vi "Load Positions.vi"(8 "error in":errorcluster) -> (0 "error out":errorcluster, 3 "positions":T1[](array[typedef]))   [LabVIEW 2020, in "Manipulator.lvlib"]
uses:
  Manipulator.lvlib
  Named Position.ctl
panel:
  out "text":string
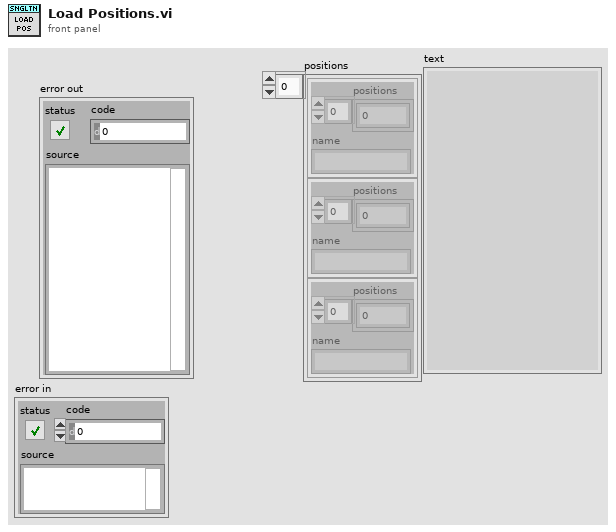
[diagram p1: front panel]
types:
  T1 = typedef "Manipulator.lvlib/Named Position.ctl" = cluster{"positions":dbl[], "name":string}
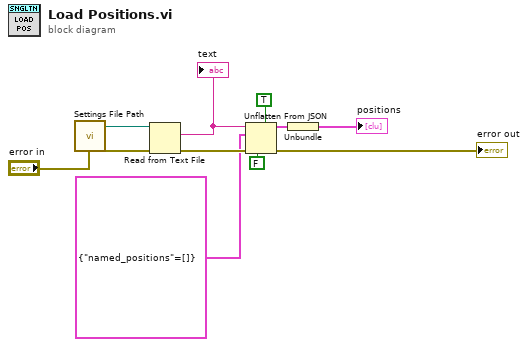
[diagram p0: block diagram]
diagram:
  n1 = call "Settings File Path.vi"() -> ("settings path"=w4:path)  [unwired: 11 in]
  n2 = Read from Text File(file (use dialog)=w4, error in="error in") -> (text=w5:string, error out=w6:errorcluster)  [unwired: 2 in, 2 out]
  "text" <- w5
  n3 = Unflatten From JSON(enable LabVIEW extensions? (T)=TRUE, JSON string=w5, type and defaults=cluster{"named_positions":T1[]} {"named_positions"=[]}, default null elements? (F)=FALSE, error in (no error)=w6) -> (value=w8:cluster{"named_positions":T1[]}, error out=→"error out":errorcluster)  [unwired: 2 in]
  n4 = Unbundle(w8) -> ("named_positions"=→"positions":T1[])
